vi "oa_FIR Preprocess Filter Kaiser-Bessel Windowed Coefficients.vi"(6 "beta":dbl=6.0, 7 "filter type":T1(ring), 8 "sampling freq: fs":dbl=1.0 format="%0.2f", 9 "low cutoff freq: fl":dbl=0.125 format="%0.2f", 10 "high cutoff freq: fh":dbl=0.45 format="%0.2f", 11 "order":i32=25 min=1) -> (0 "error":i32, 3 "FIR Windowed Coefficients":dbl[](array[numeric]) format="%.8f")   [LabVIEW 2017, in "SoundVib_RefDataProcess.lvlib"]
uses:
  <vilib>/addons/Sound and Vibration/Order Analysis/Referece Data Processing/SoundVib_RefDataProcess.lvlib
  <vilib>/Analysis/4window.llb/Kaiser-Bessel Window (DBL).vi
  <vilib>/Analysis/NI_AALBase.lvlib
  <vilib>/Analysis/NI_AALPro.lvlib
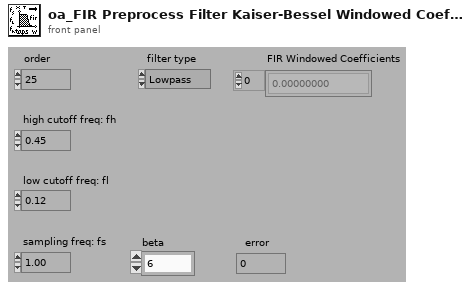
[diagram p1: front panel]
types:
  T1 = enum32{"Lowpass", "Highpass", "Bandpass", "Bandstop"}
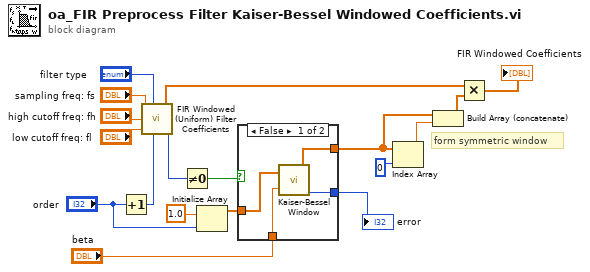
[diagram p0: block diagram]
diagram:
  # "form symmetric window"
  n1 = Increment(x="order") -> (x+1=w2:i32)
  n2 = call <vilib>:"FIR Windowed (Uniform) Filter Coefficients.vi"("sampling freq: fs"="sampling freq: fs", "filter type"="filter type", "high cutoff freq: fh"="high cutoff freq: fh", "low cutoff freq: fl"="low cutoff freq: fl", "taps"=w2) -> ("FIR Coefficients"=w10:dbl[], "error"=w5:i32)
  n3 = Not Equal To 0?(x=w5) -> (x != 0?=w3:bool)
  n4 = Initialize Array(1.0, "order") -> (w14:dbl[])
  n5 = case shown="False" w3 {
    tunnel: [w22 _] -> w16
    tunnel: w14 -> [w19 _]
    tunnel: [w21 _] -> w11
    tunnel: "beta" -> [w20 _]
    frame False {
      n6 = call-poly <vilib>:"Kaiser-Bessel Window.vi"("beta"=w20, "X"=w19) -> ("error"=w22:i32, "Windowed X"=w21:dbl[])
    }
    frame True {
    }
  }
  "error" <- w16
  n7 = Index Array(array=w11, index=0) -> (element=w12:dbl)
  n8 = Build Array (concatenate)(w11, w12) -> (w9:dbl[])
  n9 = Multiply(x=w10, y=w9) -> (x*y=→"FIR Windowed Coefficients":dbl[])
